vi "getContext.vi"(0 "subsystemMap":refnum<class "niInstr Subsystem Map v1 Host.lvclass">, 5 "instance":u8, 11 "error in":errorcluster) -> (4 "QuadEncContext":refnum<class "niInstr Instruction Framework Context v1 Host.lvclass">, 15 "error out":errorcluster)   [LabVIEW 2015, in "QuadEncInterface.lvlib"]
uses:
  QuadEncInterface.lvlib
  <instrlib>/_niInstr/Instruction Framework/v1/Host/Subsystem Map/niInstr Subsystem Map v1 Host.lvclass
  <instrlib>/_niInstr/Instruction Framework/v1/Host/Instruction Framework Context/niInstr Instruction Framework Context v1 Host.lvclass
  <instrlib>/_niInstr/Instruction Framework/v1/Host/Subsystem Map/Private/Lookup Single Context.vi
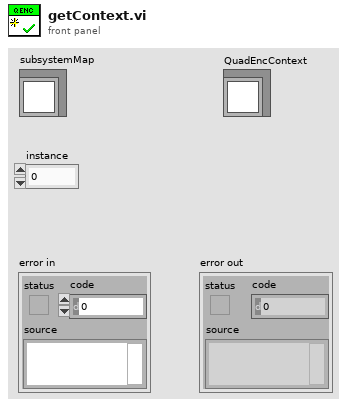
[diagram p1: front panel]
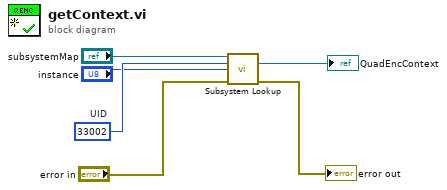
[diagram p0: block diagram]
diagram:
  w6 = u16 33002  # UID
  n1 = call-poly <instrlib>:"Subsystem Lookup.vi"("subsystem map in"="subsystemMap", "UID"=w6, "instance"="instance", "error in"="error in") -> ("context"=→"QuadEncContext":refnum<class "niInstr Instruction Framework Context v1 Host.lvclass">, "error out"=→"error out":errorcluster)  [unwired: 8 in, 2 out]
